vi "Meas Get Record Section Read MAT.vi"(5 "record id":i64, 6 "record position info":T1, 7 "sub-record id":i32, 8 "error in (no error)":errorcluster, 9 "info data in":string, 10 "full wave or sub-record? (T: full wave)":bool=TRUE, 11 "meas header path":path) -> (0 "error out":errorcluster, 1 "time vector [s]":sgl[](array[numeric]), 2 "waveform(s)":sgl[][](array[numeric]), 3 "raw MAT path":path)   [LabVIEW 2020]
doc: "Nested part of Meas Get Record Section.vi. Extracts part of wave data from MAT raw record files."
uses:
  GUI/GUI Waveform Info.ctl
  octave/infolib/Get 1D String.vi
  octave/infolib/GetI64.vi
  octave/infolib/Get 1D I64.vi
  octave/infolib/Get 2D I64.vi
  octave/infolib/Get 2D EXT.vi
  octave/infolib/Get 1D EXT.vi
  octave/infolib/infolib.lvlib
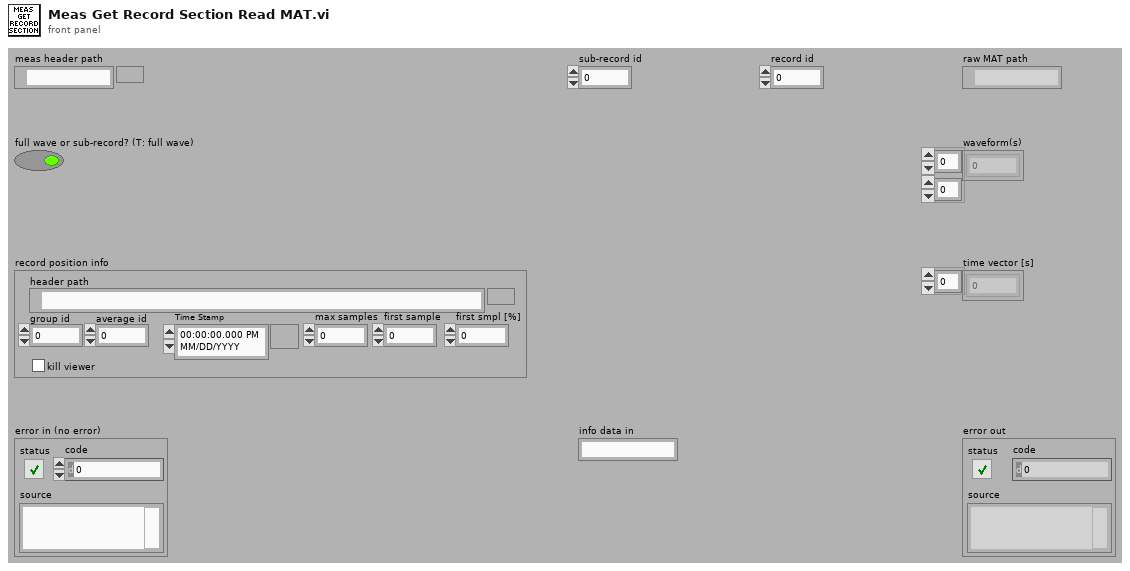
[diagram p1: front panel]
types:
  T1 = typedef "GUI Waveform Info.ctl" = cluster{"header path":path, "group id":i32, "average id":i32, "Time Stamp":timestamp, "max samples":i64, "first sample":i64, "first smpl [%]":dbl, "kill viewer":bool}
  T2 = typedef "MAT Type Representation.ctl" = enum16{"DBL", "SGL", "I32", "I16", "U16", "U8", "CDB", "CSG", "STR"}
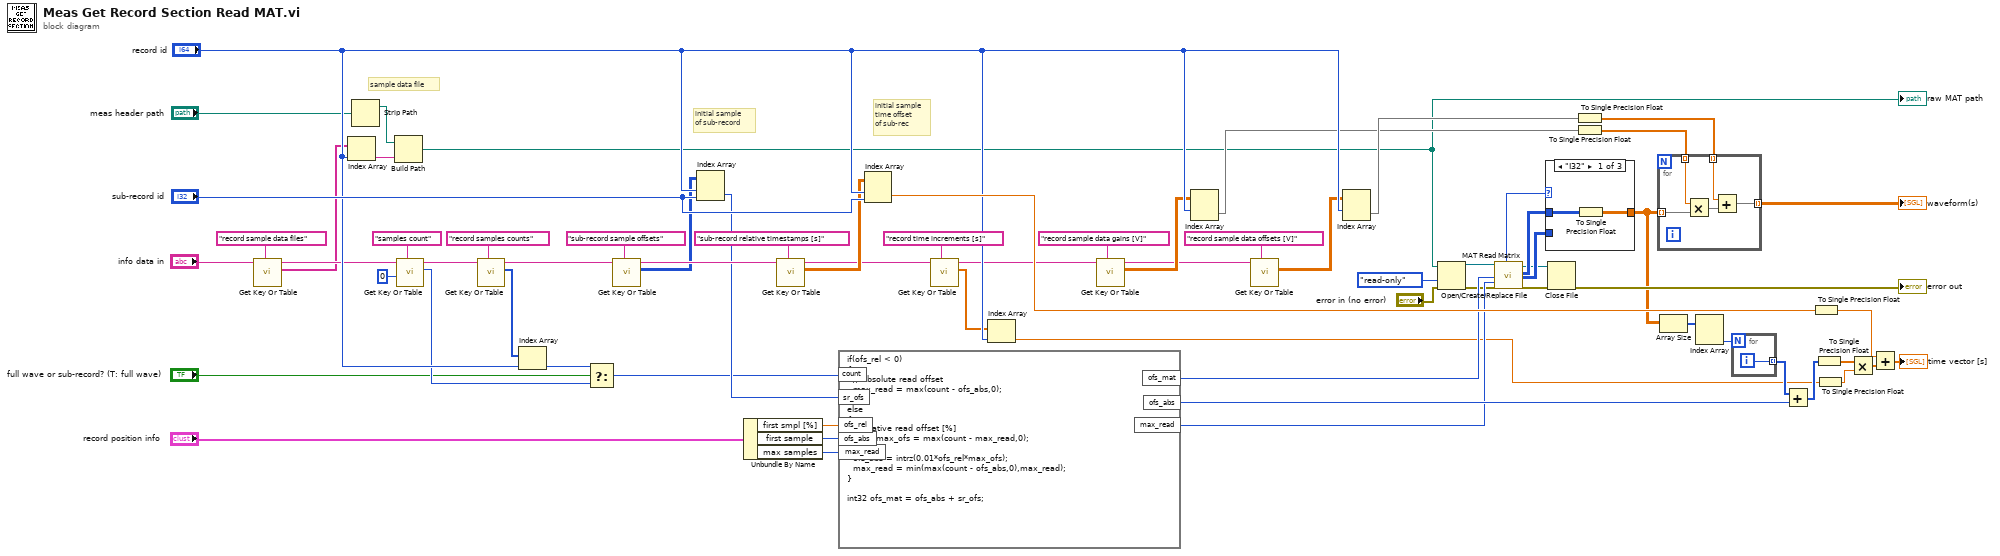
[diagram p0: block diagram]
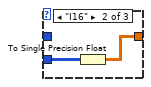
[diagram p2: hidden frame]
diagram:
  # "initial sample\ntime offset\nof sub-rec"
  # "initial sample\nof sub-record"
  # "sample data file"
  n1 = call-poly "Get Key Or Table.vi"("key description"="record sample data files", "info data"="info data in") -> ("value"=w5:string[], "info data out"=w51:string)  [unwired: 6 in, 2 out]
  n2 = Index Array(array=w5, index="record id") -> (element=w14:string)
  n3 = Strip Path(path="meas header path") -> (stripped path=w13:path)  [unwired: 1 out]
  n4 = Build Path(base path=w13, name or relative path=w14) -> (appended path=w24:path)
  "raw MAT path" <- w24
  n5 = call-poly "Get Key Or Table.vi"("key description"="samples count", "numeric"=i64 0, "info data"=w51) -> ("value"=w55:i64, "info data out"=w50:string)  [unwired: 5 in, 2 out]
  n6 = call-poly "Get Key Or Table.vi"("key description"="record samples counts", "info data"=w50) -> ("value"=w21:i64[], "info data out"=w57:string)  [unwired: 6 in, 2 out]
  n7 = Index Array(array=w21, index="record id") -> (element=w53:i64)
  n8 = Select(t=w53, s="full wave or sub-record? (T: full wave)", f=w55) -> (s? t:f=w54:i64)
  n9 = call-poly "Get Key Or Table.vi"("key description"="sub-record sample offsets", "info data"=w57) -> ("value"=w58:i64[][], "info data out"=w65:string)  [unwired: 6 in, 2 out]
  n10 = Index Array(array=w58, index (row)="record id", index (col)="sub-record id") -> (element=w59:i64)
  n11 = Unbundle By Name("record position info") -> ("first smpl [%]"=w20:dbl, "first sample"=w19:i64, "max samples"=w22:i64)
  n12 = call-poly "Get Key Or Table.vi"("key description"="sub-record relative timestamps [s]", "info data"=w65) -> ("value"=w66:ext[][], "info data out"=w64:string)  [unwired: 6 in, 2 out]
  n13 = formula code="if(ofs_rel < 0)\n{\n  // absolute read offset\n  max_read = max(count - ofs_abs,0);\n}\nelse\n{\n  // relative read offset [%]\n  int32 max_ofs = max(count - max_read,0);\n  \n  ofs_abs = intrz(0.01*ofs_rel*max_ofs);\n  max_read = min(max(count - ofs_abs,0),max_read);\n}\n\nint32 ofs_mat = ofs_abs + sr_ofs;"("max_read"=w22, "count"=w54, "ofs_abs"=w19, "ofs_rel"=w20, "sr_ofs"=w59) -> ("ofs_abs"=w48:i64, "max_read"=w23:i64, "ofs_mat"=w62:i32)
  n14 = Index Array(array=w66, index (row)="record id", index (col)="sub-record id") -> (element=w69:ext)
  n15 = call-poly "Get Key Or Table.vi"("key description"="record time increments [s]", "info data"=w64) -> ("value"=w40:ext[], "info data out"=w35:string)  [unwired: 6 in, 2 out]
  n16 = Index Array(array=w40, index="record id") -> (element=w3:ext)
  n17 = call-poly "Get Key Or Table.vi"("key description"="record sample data gains [V]", "info data"=w35) -> ("value"=w10:ext[][], "info data out"=w9:string)  [unwired: 6 in, 2 out]
  n18 = Index Array(array=w10, index (row)="record id") -> (element=w30:ext[])  [unwired: 1 in]
  n19 = call-poly "Get Key Or Table.vi"("key description"="record sample data offsets [V]", "info data"=w9) -> ("value"=w11:ext[][])  [unwired: 6 in, 3 out]
  n20 = Index Array(array=w11, index (row)="record id") -> (element=w31:ext[])  [unwired: 1 in]
  n21 = Open/Create/Replace File(file path (use dialog)=w24, error in="error in (no error)", access (0:read/write)=enum16{"read/write", "read-only", "write-only"}."read-only") -> (refnum out=w17:refnum<file>, error out=w16:errorcluster)  [unwired: 3 in, 1 out]
  n22 = call "MAT Read Matrix.vi"("Ref Num"=w17, "first matrix column (0: first one)"=w62, "maximum matrix columns (-1: all)"=w23, "Error In"=w16) -> ("Representation"=w27:T2, "Dup Ref Num"=w26:refnum<file>, "I32"=w28:i32[][], "I16"=w29:i16[][], "error out"=w25:errorcluster)  [unwired: 3 in, 8 out]
  n23 = case shown="\"I32\"" w27 {
    tunnel: w28 -> [w71 _ _]
    tunnel: w29 -> [_ w73 _]
    tunnel: [w70 w72 _] -> w36
    frame "I32" {
      n24 = To Single Precision Float(number=w71) -> (single precision float=w70:sgl[][])
    }
    frame "I16" {
      n25 = To Single Precision Float(number=w73) -> (single precision float=w72:sgl[][])
    }
    frame Default {
    }
  }
  n26 = Close File(refnum=w26, error in=w25) -> (error out=→"error out":errorcluster)  [unwired: 1 out]
  n27 = To Single Precision Float(number=w31) -> (single precision float=w32:sgl[])
  n28 = To Single Precision Float(number=w30) -> (single precision float=w33:sgl[])
  n29 = for {
    tunnel: w36 -> [w78] mode=indexing
    tunnel: w33 -> [w77] mode=indexing
    tunnel: w32 -> [w75] mode=indexing
    tunnel: [w74] -> w43 mode=indexing
    n30 = Multiply(x=w77, y=w78) -> (x*y=w76:sgl[])
    n31 = Add(x=w75, y=w76) -> (x+y=w74:sgl[])
  }
  "waveform(s)" <- w43
  n32 = Array Size(array=w36) -> (size(s)=w37:i32[])
  n33 = Index Array(array=w37) -> (element #2=w38:i32)  [unwired: 2 in, 1 out]
  n34 = for {
    N: w38 -> [_]
    tunnel: [w79] -> w46 mode=indexing
    i -> [w79]
  }
  n35 = Add(x=w46, y=w48) -> (x+y=w47:i64[])
  n36 = To Single Precision Float(number=w69) -> (single precision float=w1:sgl)
  n37 = To Single Precision Float(number=w47) -> (single precision float=w39:sgl[])
  n38 = To Single Precision Float(number=w3) -> (single precision float=w45:sgl)
  n39 = Multiply(x=w39, y=w45) -> (x*y=w44:sgl[])
  n40 = Add(x=w1, y=w44) -> (x+y=→"time vector [s]":sgl[])
